vi "Framework Status.Create.vi"(8 "error in (no error)":errorcluster) -> (0 "error out":errorcluster, 3 "Framework Status":refnum<class "Framework Status.lvclass">)   [LabVIEW 2017, in "DSF Core.lvlib" / "Framework Status.lvclass"]
uses:
  Framework Status.lvclass
  Framework Status.lvclass/Framework Status.ctl
  Framework Performance.lvclass
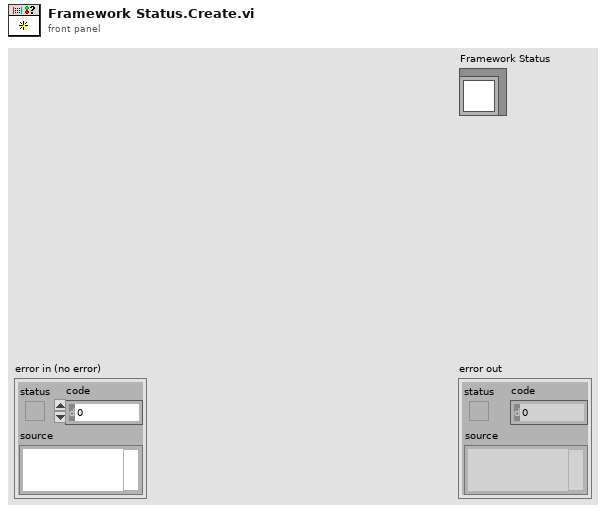
[diagram p1: front panel]
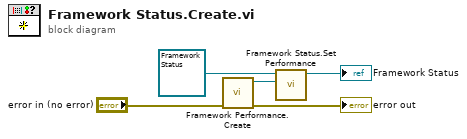
[diagram p0: block diagram]
diagram:
  n1 = call "Framework Performance.Create.vi"("error in (no error)"="error in (no error)") -> ("error out"=→"error out":errorcluster, "Framework Performance"=w3:refnum<class "Framework Performance.lvclass">)  [unwired: 9 in]
  n2 = call "Framework Status.Set Performance.vi"("Framework Performance"=w3, "Framework Status in"=refnum<class "Framework Status.lvclass"> refnum) -> ("Framework Status out"=→"Framework Status":refnum<class "Framework Status.lvclass">)  [unwired: 9 in]
